vi "calcMirrorAuth.vi"(8 "error in (no error)":errorcluster, 9 "Num of Bending Mode":i32=20, 10 "Subsystem":T1={"Mirror"="M1M3", "Actuatro Force File"="M1M3_1um_156_force.DAT"}, 11 "OptCtrl in":refnum<class "OptCtrl.lvclass">) -> (0 "error out":errorcluster, 2 "Authority (1 N RMS)":dbl[](array[numeric]), 3 "OptCtrl out":refnum<class "OptCtrl.lvclass">)   [LabVIEW 2016, in "OptCtrl.lvclass"]
doc: "Calculate the distribution of control authority of mirror."
uses:
  OptCtrl.lvclass
  OptCtrl.lvclass/OptCtrl.ctl
  Utility/getSubArray2D.vi
  <vilib>/Analysis/NI_AALBase.lvlib
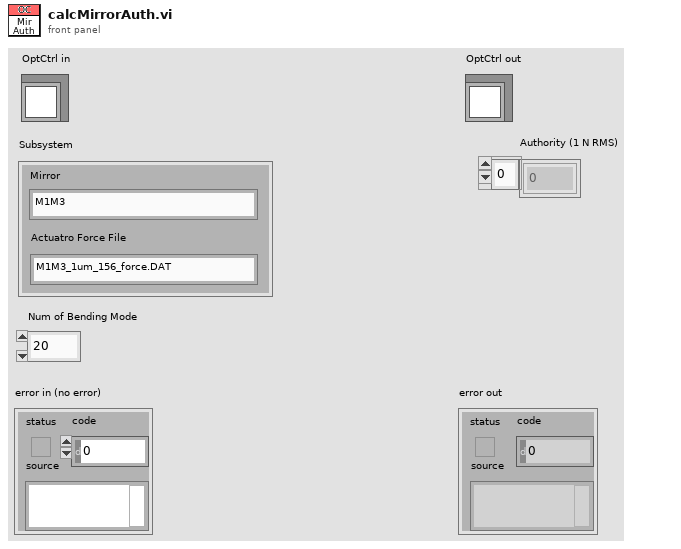
[diagram p1: front panel]
types:
  T1 = cluster{"Mirror":string, "Actuatro Force File":string}
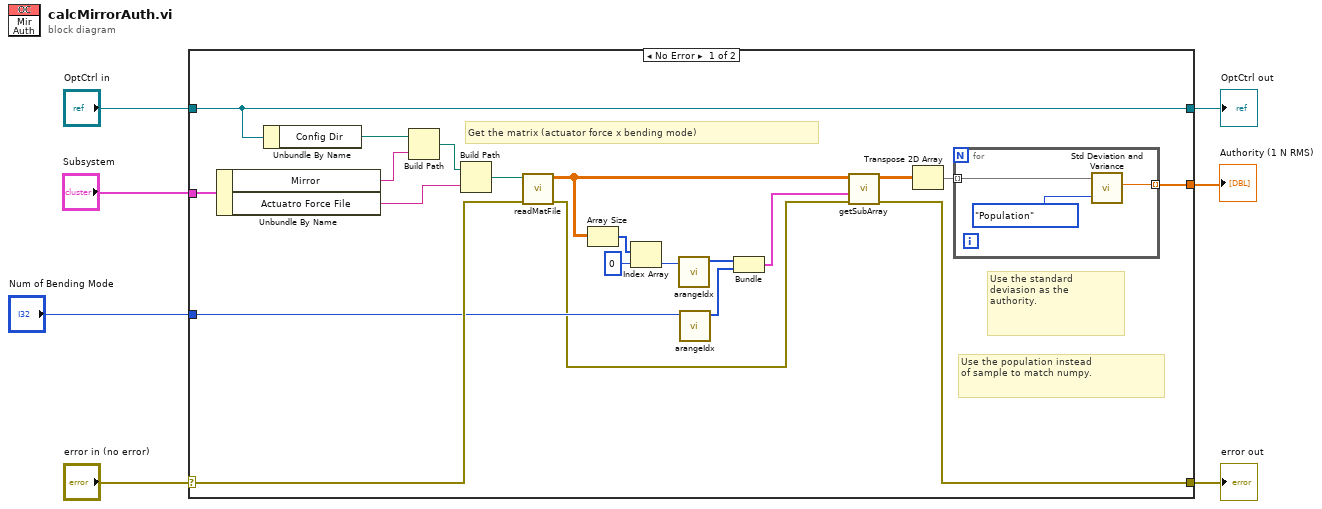
[diagram p0: block diagram]
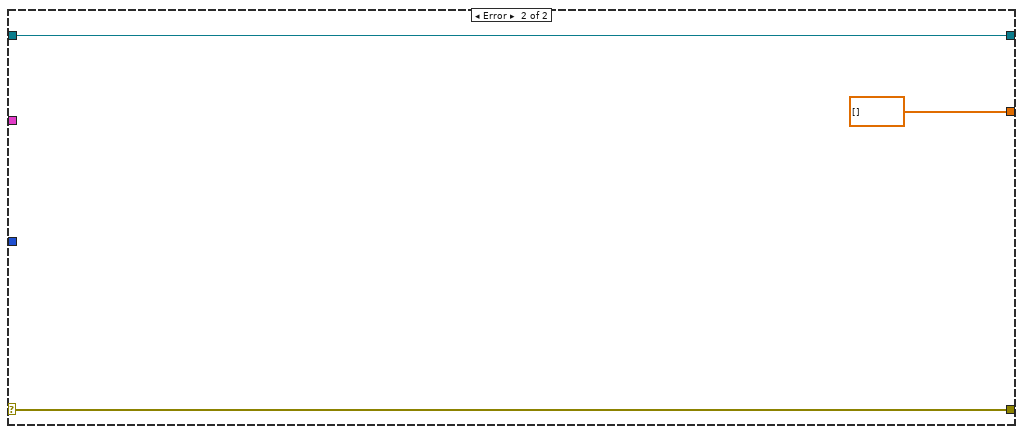
[diagram p2: hidden frame]
diagram:
  n1 = case shown="No Error" "error in (no error)" {
    selector: "error in (no error)" -> [w21 w34]
    tunnel: [w15 w34] -> w6
    tunnel: [w27 w33] -> w4
    tunnel: "OptCtrl in" -> [w27 w33]
    tunnel: "Subsystem" -> [w28 _]
    tunnel: "Num of Bending Mode" -> [w17 _]
    tunnel: [w8 dbl[] []] -> w1
    frame No Error {
      # "Use the population instead\nof sample to match numpy."
      # "Use the standard \ndeviasion as the \nauthority."
      # "Get the matrix (actuator force x bending mode)"
      n2 = Unbundle By Name(w28) -> ("Mirror"=w25:string, "Actuatro Force File"=w23:string)
      n3 = Unbundle By Name(w27) -> ("Config Dir"=w26:path)
      n4 = Build Path(base path=w26, name or relative path=w25) -> (appended path=w24:path)
      n5 = Build Path(base path=w24, name or relative path=w23) -> (appended path=w22:path)
      n6 = call "readMatFile.vi"("error in (no error)"=w21, "Path"=w22) -> ("error out"=w14:errorcluster, "Matrix"=w16:dbl[][])  [unwired: 8 in]
      n7 = Array Size(array=w16) -> (size(s)=w20:i32[])
      n8 = Index Array(array=w20, index=0) -> (element=w18:i32)
      n9 = call "arangeIdx.vi"("Number"=w18) -> ("Idx Array"=w13:i32[])  [unwired: 10 in]
      n10 = call "arangeIdx.vi"("Number"=w17) -> ("Idx Array"=w12:i32[])  [unwired: 10 in]
      n11 = Bundle("Idx Array"=w13, "Idx Array"=w12) -> (w11:cluster{"Idx Array":i32[], "Idx Array":i32[]})  [unwired: 1 in]
      n12 = call-poly "getSubArray.vi"("error in (no error)"=w14, "Index Array Cluster"=w11, "2D Array"=w16) -> ("error out"=w15:errorcluster, "Sub-Array"=w10:dbl[][])  [unwired: 7 in]
      n13 = Transpose 2D Array(2D array=w10) -> (transposed array=w9:dbl[][])
      n14 = for {
        tunnel: w9 -> [w31] mode=indexing
        tunnel: [w30] -> w8 mode=indexing
        n15 = call <vilib>:"Std Deviation and Variance.vi"("X"=w31, "Weighting (Sample)"=enum16{"Sample", "Population"}."Population") -> ("standard deviation"=w30:dbl)  [unwired: 2 out]
      }
    }
    frame Error {
    }
  }
  "error out" <- w6
  "OptCtrl out" <- w4
  "Authority (1 N RMS)" <- w1
